vi "Write WaveGenerator.vi"(8 "error in (no error)":errorcluster, 10 "WaveGenerator.lvclass":refnum<class "WaveGenerator.lvclass">, 11 "UserInterface in":refnum<class "UserInterface.lvclass">) -> (0 "error out":errorcluster, 3 "UserInterface out":refnum<class "UserInterface.lvclass">)   [LabVIEW 2021, in "UserInterface.lvclass"]
uses:
  UserInterface.lvclass
  WaveGenerator/WaveGenerator.lvclass
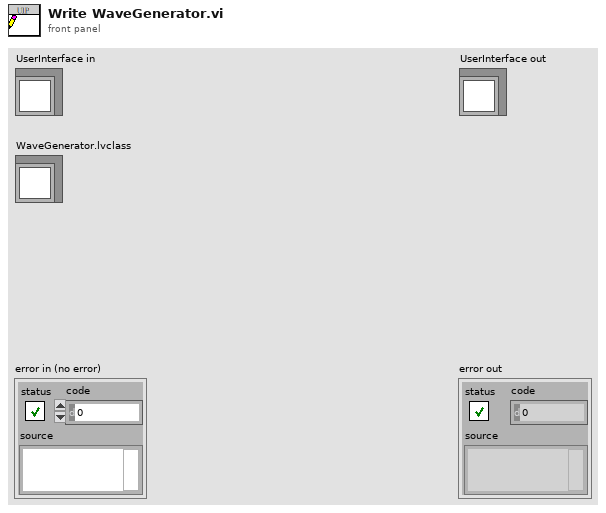
[diagram p1: front panel]
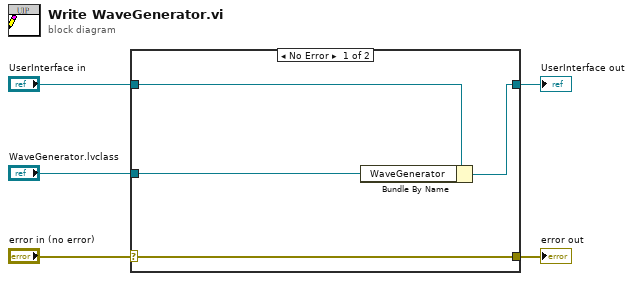
[diagram p0: block diagram]
diagram:
  n1 = case shown="No Error" "error in (no error)" {
    selector: "error in (no error)" -> [w9 w10]
    tunnel: [w9 w10] -> w4
    tunnel: [w7 w11] -> w2
    tunnel: "UserInterface in" -> [w8 w11]
    tunnel: "WaveGenerator.lvclass" -> [w6 _]
    frame No Error {
      n2 = Bundle By Name(cluster=w8, "WaveGenerator"=w6) -> (w7:refnum<class "UserInterface.lvclass">)
    }
    frame Error {
    }
  }
  "error out" <- w4
  "UserInterface out" <- w2
